vi "Open Options to Bit Mask.vi"(1 "Options":T1) -> (0 "Bit Mask":u32)   [LabVIEW 2018, in "Toolkit.lvlib" / "SFTP File.lvclass"]
doc: "Converts SFTP File open options to a C-style bit mask."
uses:
  SFTP File.lvclass
  Type Definitions/Open Options.ctl
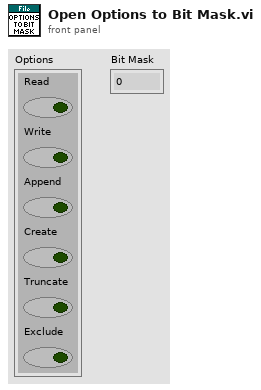
[diagram p1: front panel]
types:
  T1 = typedef "Toolkit.lvlib/SFTP File.lvclass/Open Options.ctl" = cluster{"Read":bool, "Write":bool, "Append":bool, "Create":bool, "Truncate":bool, "Exclude":bool}
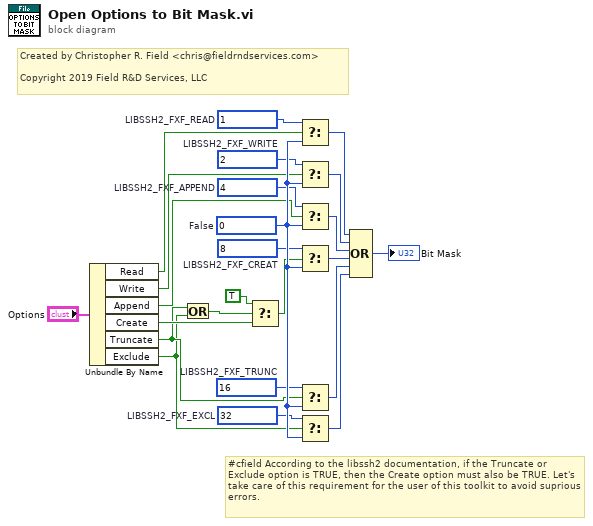
[diagram p0: block diagram]
diagram:
  w18 = u32 32  # LIBSSH2_FXF_EXCL
  w19 = u32 16  # LIBSSH2_FXF_TRUNC
  w20 = u32 8  # LIBSSH2_FXF_CREAT
  w21 = u32 4  # LIBSSH2_FXF_APPEND
  w22 = u32 2  # LIBSSH2_FXF_WRITE
  w23 = u32 1  # LIBSSH2_FXF_READ
  w24 = u32 0  # False
  # "#cfield According to the libssh2 documentation, if the Truncate or Exclude option is TRUE, then the Create option must also be TRUE. Let's take care of this requirement for the user of this toolkit to avoid suprious errors."
  # "Created by Christopher R. Field <chris@fieldrndservices.com>\n\nCopyright 2019 Field R&D Services, LLC"
  n1 = Unbundle By Name("Options") -> ("Read"=w16:bool, "Write"=w15:bool, "Append"=w14:bool, "Create"=w5:bool, "Truncate"=w4:bool, "Exclude"=w3:bool)
  n2 = Or(x=w4, y=w3) -> (x .or. y?=w2:bool)
  n3 = Select(t=TRUE, s=w2, f=w5) -> (s? t:f=w1:bool)
  n4 = Select(t=w23, s=w16, f=w24) -> (s? t:f=w13:u32)
  n5 = Select(t=w22, s=w15, f=w24) -> (s? t:f=w12:u32)
  n6 = Select(t=w21, s=w14, f=w24) -> (s? t:f=w11:u32)
  n7 = Select(t=w20, s=w1, f=w24) -> (s? t:f=w10:u32)
  n8 = Select(t=w19, s=w4, f=w24) -> (s? t:f=w9:u32)
  n9 = Select(t=w18, s=w3, f=w24) -> (s? t:f=w8:u32)
  n10 = Compound Arithmetic op=OR(w13, w12, w11, w10, w9, w8) -> (→"Bit Mask":u32)
